vi "ReplaceAllSimilar.vi"(9 "min value":dbl, 10 "Magnitude array":dbl[](array[numeric]), 11 "min index(es)":i32) -> (3 "Magnitude array 2":dbl[](array[numeric]))   [LabVIEW 2014]
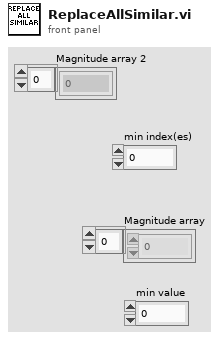
[diagram p1: front panel]
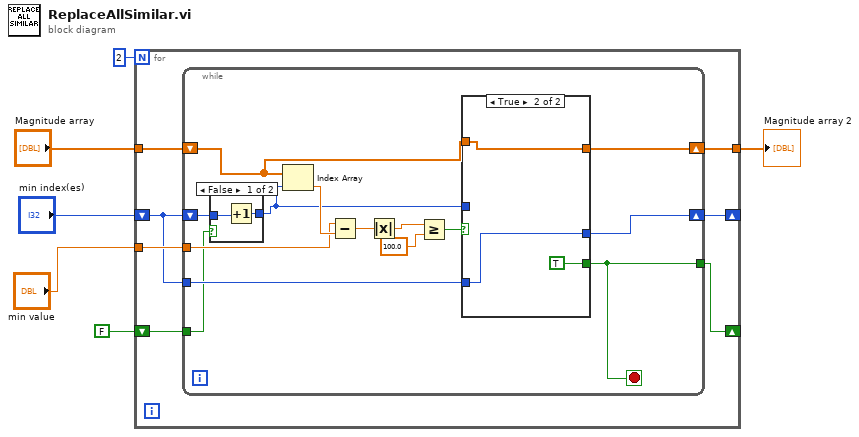
[diagram p0: block diagram]
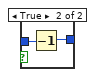
[diagram p2: hidden frame]
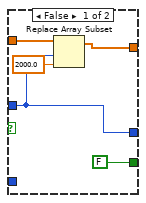
[diagram p3: hidden frame]
diagram:
  n1 = for {
    N: 2 -> [_]
    tunnel: "Magnitude array" -> [w13]
    tunnel: "min value" -> [w12]
    shift-right: [w10] -> _
    shift-left: "min index(es)" -> [w11]
    shift-right: [w8] -> _
    shift-left: FALSE -> [w9]
    tunnel: [w7] -> w1
    n2 = while {
      shift-right: [w21] -> w10
      shift-left: w11 -> [w17]
      tunnel: w12 -> [w26]
      tunnel: w11 -> [w20]
      shift-right: [w18] -> w7
      shift-left: w13 -> [w19]
      tunnel: w9 -> [w15]
      tunnel: [w14] -> w8
      stop <- w14 stop-if-true
      n3 = case shown="False" w15 {
        tunnel: w17 -> [w29 w31]
        tunnel: [w28 w30] -> w16
        frame False {
          n4 = Increment(x=w29) -> (x+1=w28:i32)
        }
        frame True {
          n5 = Decrement(x=w31) -> (x-1=w30:i32)
        }
      }
      n6 = Index Array(array=w19, index=w16) -> (element=w27:dbl)
      n7 = Subtract(x=w26, y=w27) -> (x-y=w25:dbl)
      n8 = Absolute Value(x=w25) -> (abs(x)=w24:dbl)
      n9 = Greater Or Equal?(x=w24, y=100.0) -> (x >= y?=w22:bool)
      n10 = case shown="True" w22 {
        tunnel: w16 -> [w33 _]
        tunnel: [w33 w39] -> w21
        tunnel: w20 -> [_ w39]
        tunnel: w19 -> [w36 w38]
        tunnel: [w34 w38] -> w18
        tunnel: [FALSE TRUE] -> w14
        frame False {
          n11 = Replace Array Subset(array=w36, new element=2000.0 ("new element/subarray"), index=w33) -> (w34:dbl[])
        }
        frame True {
        }
      }
    }
  }
  "Magnitude array 2" <- w1
